vi "ShutdownDaily.vi"(2 "Error In":errorcluster) -> (0 "ErrorOut":errorcluster)   [LabVIEW 2014]
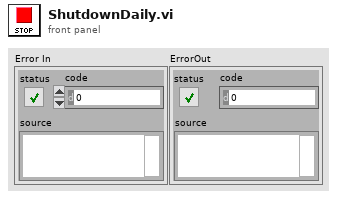
[diagram p1: front panel]
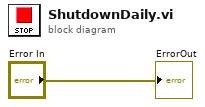
[diagram p0: block diagram]
diagram:
  "ErrorOut" <- "Error In"
